vi "AG33XXX.use external amplitude modulation.vi"(0 "i ref in":refnum<vi>, 3 "ms timeout (10000)":i32=10000, 5 "error in (no error)":errorcluster) -> (14 "i ref out":refnum<vi>, 17 "timed out":bool, 19 "error out":errorcluster)   [LabVIEW 2014, in "AG33XXX.lvlib"]
doc: "Enables external amplitude modulation of the device."
uses:
  AG33XXX.lvlib
  CS_Core/CSApplicationBaseClasses/AFGBase/AFGBase.serviceType.ctl
  CS_Core/CSApplicationBaseClasses/AFGBase/AFGBase.directionType.ctl
  CSlibraries/UtilityLib/UtilityLib.valueStatus.ctl
  CS_Core/CSApplicationBaseClasses/AFGBase/AFGBase.waveformType.ctl
  CS_Core/CSApplicationBaseClasses/DeviceBase/DeviceBase.lvlib
  CS_Core/CSApplicationBaseClasses/AFGBase/AFGBase.lvlib
  CSlibraries/UtilityLib/UtilityLib.lvlib
  instr.lib/agilent_33xxx_series/Agilent 33XXX Series/Agilent 33XXX Series.lvlib
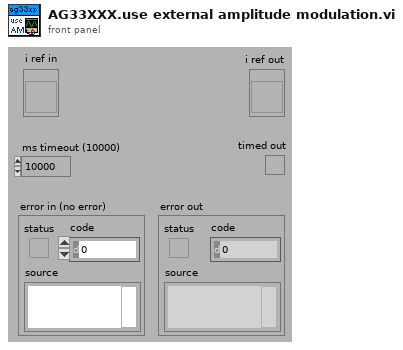
[diagram p1: front panel]
types:
  T1 = typedef "AFGBase.lvlib/AFGBase.waveformType.ctl" = enum16{"sine", "square", "ramp", "pulse", "noise", "DC", "arbitrary", "triangle", "ramp_up", "ramp_down", "amplitude modulation"}
  T2 = typedef "UtilityLib.lvlib/UtilityLib.valueStatus.ctl" = enum16{"no info available", "stand by/off", "on", "warning", "alarm/malfunction", "not implemented", "user action required", "important information", "system default", "control default", "indicator default", "button default"}
  T3 = typedef "AFGBase.lvlib/AFGBase.directionType.ctl" = enum16{"unknown", "update actual value", "update nominal value", "update both"}
  T4 = typedef "AFGBase.lvlib/AFGBase.serviceType.ctl" = enum16{"frequency", "amplitude", "phase", "DCOffset", "enableOutput", "trigger", "waveformType"}
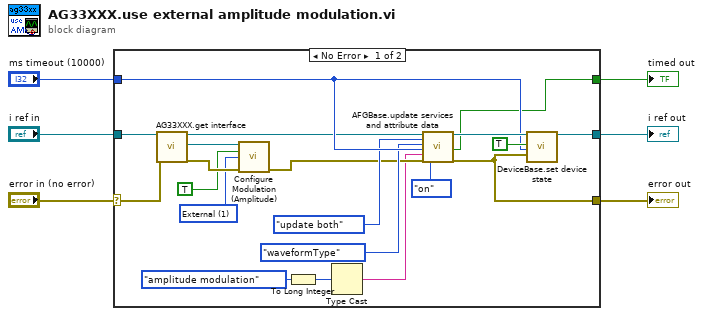
[diagram p0: block diagram]
diagram:
  n1 = case shown="No Error" "error in (no error)" {
    selector: "error in (no error)" -> [w17 w27]
    tunnel: [w26 w28] -> w6
    tunnel: "ms timeout (10000)" -> [w22 _]
    tunnel: "i ref in" -> [w18 w28]
    tunnel: [w23 w27] -> w2
    tunnel: [w7 _] -> w1
    frame No Error {
      w11 = 1 items=["Internal", "External"] ("AM Source (0: Internal)")
      n2 = call "AG33XXX.get interface.vi"("i ref in"=w18, "error in (no error)"=w17) -> ("i ref out"=w16:refnum<vi>, "interface"=w14:refnum<visa-resource-name>, "error out"=w15:errorcluster)  [unwired: 15 in]
      n3 = call "Configure Modulation (Amplitude).vi"("VISA resource name"=w14, "Enable Amplitude Modulation (True)"=TRUE, "AM Source (0: Internal)"=w11, "error in (no error)"=w15) -> ("error out"=w13:errorcluster)  [unwired: 10 in, 1 out]
      n4 = To Long Integer(number=AFGBase.waveformType."amplitude modulation" ("waveformType")) -> (32bit integer=w8:i32)
      n5 = Type Cast(x=w8) -> (*(type *) &x=w10:string)  [unwired: 1 in]
      n6 = call "AFGBase.update services and attribute data.vi"("i ref in"=w16, "direction"=AFGBase.directionType."update both", "service"=AFGBase.serviceType."waveformType", "ms timeout (10000)"=w22, "value"=w10, "error in (no error)"=w13, "quality"=UtilityLib.valueStatus."on") -> ("i ref out"=w24:refnum<vi>, "timed out"=w7:bool, "error out"=w23:errorcluster)  [unwired: 10 in]
      n7 = call "DeviceBase.set device state.vi"("i ref in"=w24, "implicit"=TRUE, "ms timeout (10000)"=w22, "device error"=w23) -> ("i ref out"=w26:refnum<vi>)  [unwired: 13 in, 2 out]
    }
    frame Error {
    }
  }
  "error out" <- w2
  "i ref out" <- w6
  "timed out" <- w1
